vi "Guitar A440.vi"() -> ()   [LabVIEW 2012]
uses:
  <vilib>/ptbypt/NI_PtbyPt.lvlib
panel:
  in  "stop":bool
  in  "P":i32(slide) scale=0.0..10.0
  out "Waveform Graph":waveform(dbl)(graph)
  in  "N":i32(slide) scale=0.0..10.0
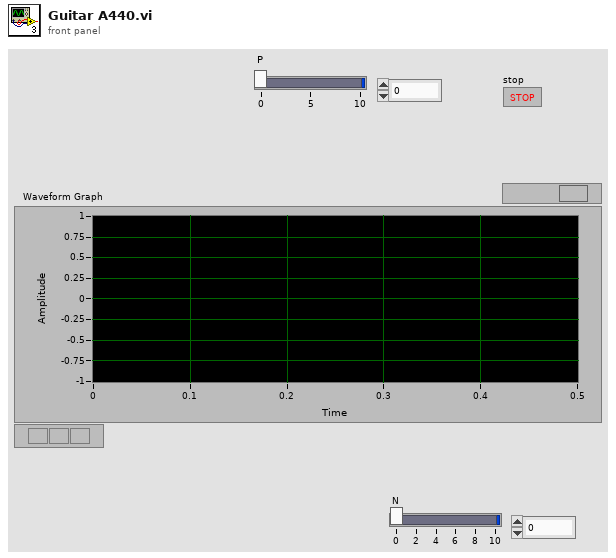
[diagram p1: front panel]
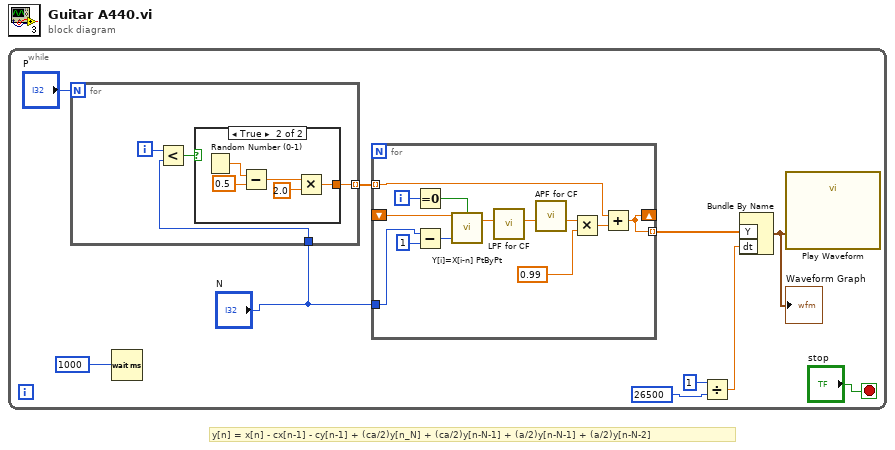
[diagram p0: block diagram]
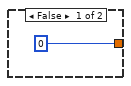
[diagram p2: hidden frame]
diagram:
  # "y[n] = x[n] - cx[n-1] - cy[n-1] + (ca/2)y[n_N] + (ca/2)y[n-N-1] + (a/2)y[n-N-1] + (a/2)y[n-N-2]"
  n1 = while {
    stop <- "stop" stop-if-true
    n2 = for {
      N: "P" -> [_]
      tunnel: [w14] -> w9 mode=indexing
      tunnel: "N" -> [w11]
      i -> [w12]
      n3 = Less?(x=w12, y=w11) -> (x < y?=w13:bool)
      n4 = case shown="True" w13 {
        tunnel: [0 w18] -> w14
        frame False {
        }
        frame True {
          n5 = Random Number (0-1)() -> (number: 0 to 1=w20:dbl)
          n6 = Subtract(x=w20, y=0.5) -> (x-y=w17:dbl)
          n7 = Multiply(x=w17, y=2.0) -> (x*y=w18:dbl)
        }
      }
    }
    n8 = Wait (ms)(milliseconds to wait=1000) -> ()  [unwired: 1 out]
    n9 = for {
      shift-right: [w28] -> _
      shift-left: _ -> [w30]
      tunnel: [w28] -> w7 mode=indexing
      tunnel: w9 -> [w29] mode=indexing
      tunnel: "N" -> [w26]
      i -> [w32]
      n10 = Equal To 0?(x=w32) -> (x = 0?=w31:bool)
      n11 = Subtract(x=w26, y=1) -> (x-y=w25:i32)
      n12 = call <vilib>:"Y[i]=X[i-n] PtByPt.vi"("initialize"=w31, "shifts: n"=w25, "x"=w30) -> ("shifted x"=w27:dbl)  [unwired: 1 in, 1 out]
      n13 = call "LPF for CF.vi"("Numeric"=w27) -> ("Numeric 2"=w23:dbl)  [unwired: 10 in]
      n14 = call "APF for CF.vi"("Input Signal Sample (q)"=w23) -> ("Output Signal Sample (r)"=w22:dbl)  [unwired: 8 in]
      n15 = Multiply(x=w22, y=0.99) -> (x*y=w33:dbl)
      n16 = Add(x=w29, y=w33) -> (x+y=w28:dbl)
    }
    n17 = Divide(x=1, y=26500) -> (x/y=w4:dbl)
    n18 = Bundle By Name("Y"=w7, "dt"=w4) -> (w8:waveform(dbl))  [unwired: 1 in]
    "Waveform Graph" <- w8
    n19 = call "Play Waveform"("Data"=w8) -> ()  [unwired: 18 in, 1 out]
  }
